vi "PVCAM_InitSeq.vi"(8 "error in (no error)":errorcluster) -> (0 "error out":errorcluster, 2 "return":i16)   [LabVIEW 2021]
uses:
  pvcam64.dll
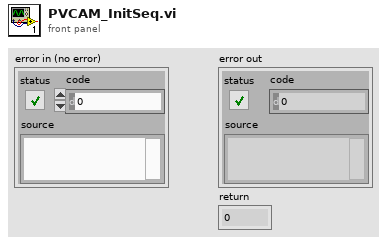
[diagram p1: front panel]
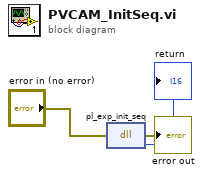
[diagram p0: block diagram]
diagram:
  n1 = dll-call lib="pvcam64.dll" fn="pl_exp_init_seq"(error in="error in (no error)") -> (error out=→"error out":errorcluster, "return type"=→"return":i16)  [unwired: 2 in, 1 out]
